vi "DSF.Engine.Framework.Rx.Async.vi"(8 "error in (no error)":errorcluster, 11 "Framework in":refnum<class "DSF.Engine.Framework.lvclass">) -> (0 "error out":errorcluster, 3 "Framework out":refnum<class "DSF.Engine.Framework.lvclass">)   [LabVIEW 2017, in "DSF.Engine.lvlib" / "DSF.Engine.Framework.lvclass"]
uses:
  DSF.Engine.Framework.lvclass
  DSF.Engine.Framework.lvclass/DSF.Engine.Framework.ctl
  Plugin/DSF.Engine.Plugin.lvclass/DSF.Engine.Plugin.ctl
  Timing/DSF.Engine.Timing.lvclass/DSF.Engine.Timing.ctl
  Transfer/DSF.Engine.Transfer Group.lvclass/DSF.Engine.Transfer Group.ctl
  Transfer/DSF.Engine.Transfer.lvclass/DSF.Engine.Transfer.ctl
  <vilib>/National Instruments/Memory Manager/Classes/Pointer/Memory.Pointer.lvclass/Memory.Pointer.ctl
  Thread Pool/DSF.Engine.Pool.lvclass/DSF.Engine.Pool.ctl
  Transceiver/DSF.Engine.Transceiver Thread.lvclass/DSF.Engine.Transceiver Thread.ctl
  Interface/DSF.Engine.Interface.lvclass/DSF.Engine.Interface.ctl
  Plugin/DSF.Engine.Plugin.Get Async Rx Transfer Groups.vi
  Timing/DSF.Engine.Timing.Get Iteration.vi
  Plugin/DSF.Engine.Plugin.Get Timing.vi
  Transfer/DSF.Engine.Transfer Group.Is Active.vi
  Plugin/DSF.Engine.Plugin.Rx.Transfer Group.Send.vi
  Plugin/DSF.Engine.Plugin.Rx.Transfer Group.Retrieve Async.vi
  Plugin/DSF.Engine.Plugin.Transfer Group.Iteration.Increment.vi
  Plugin/DSF.Engine.Plugin.Rx.Transfer Group.Move Data.vi
  Plugin/DSF.Engine.Plugin.Set Async Rx Transfer Groups.vi
  Timing/DSF.Engine.Timing.Is Active Cycle.vi
  Transfer/DSF.Engine.Transfer Group.Get Timing.vi
  Plugin/DSF.Engine.Plugin.Transceiver Thread.Obtain.vi
  Transceiver/DSF.Engine.Transceiver Thread.Command.Transfer Group.vi
  Transfer/DSF.Engine.Transfer Group.Retrieve from FIFO.vi
  Transfer/DSF.Engine.Transfer Group.Increment Iteration.vi
  Transfer/DSF.Engine.Transfer Group.Move Channels to Engine.vi
  Timing/DSF.Engine.Timing.Get Decimation.vi
  Timing/DSF.Engine.Timing.Get Offset.vi
  Thread Pool/DSF.Engine.Pool.ID.Obtain ID from Pool.vi
  Plugin/DSF.Engine.Plugin.Get Thread ID Pool.vi
  Plugin/DSF.Engine.Plugin.Get Transceiver Thread.vi
  Transceiver/DSF.Engine.Transceiver Thread.Get Interface.vi
  Interface/DSF.Engine.Interface.Transceiver.Write.vi
  Interface/DSF.Engine.Interface.Transceiver.Write.Command.vi
  Transfer/DSF.Engine.Transfer Group.Get ID.vi
  Transfer/DSF.Engine.Transfer Group.Return FIFO.Read.vi
  Transfer/DSF.Engine.Transfer Group.Set Timing.vi
  Timing/DSF.Engine.Timing.Iteration.Increment.vi
  Transfer/DSF.Engine.Transfer Group.Get Transfers.vi
  <vilib>/National Instruments/Memory Manager/Classes/Pointer/Memory.Pointer.Copy All.vi
  Transfer/DSF.Engine.Transfer.Get Inline Buffer.vi
  Transfer/DSF.Engine.Transfer.Get Intermediate Buffer.vi
  Thread Pool/DSF.Engine.Pool.Read FIFO.vi
  Interface/DSF.Engine.Interface.RT FIFO.Write.16B.vi
  Interface/DSF.Engine.Interface.Get Command FIFO.vi
  Transfer/DSF.Engine.Transfer Group.Get Return FIFO.vi
  Timing/DSF.Engine.Timing.Set Iteration.vi
  <vilib>/National Instruments/Memory Manager/Classes/Pointer/Memory.Pointer.Get Size.vi
  <vilib>/National Instruments/Memory Manager/Classes/Pointer/Memory.Pointer.Copy.vi
  Thread Pool/DSF.Engine.Pool.Get FIFO.vi
  <vilib>/National Instruments/Memory Manager/Classes/Pointer/Memory.Pointer.Copy.No Check.vi
  <vilib>/National Instruments/Memory Manager/Classes/Pointer/Memory.Pointer.Parameter Check.Subset.vi
  <vilib>/National Instruments/Memory Manager/Classes/Pointer/Memory.Pointer.Parameter Check.Null Pointer.vi
  <vilib>/National Instruments/Memory Manager/Classes/Pointer/Memory.Pointer.Get Address.vi
  <vilib>/National Instruments/Memory Manager/Classes/Pointer/Memory.Pointer.Errors.vi
  <vilib>/National Instruments/Memory Manager/Classes/Pointer/Memory.Pointer.Errors.Out of Bounds.vi
  <vilib>/National Instruments/Memory Manager/Classes/Pointer/Memory.Pointer.Errors.Null Pointer.vi
  <vilib>/NI/Static Error Handling/VIs/Static Error Handling.Source Buffer.Write.String.vi
  <vilib>/National Instruments/Memory Manager/Classes/Pointer/Memory.Pointer.Errors.Write Pointer Size.vi
  <vilib>/National Instruments/Memory Manager/Classes/Pointer/Memory.Pointer.Errors.Create Error.vi
  <vilib>/NI/Static Error Handling/VIs/Static Error Handling.Source Buffer.Write.Numeric.Scalar.Base10.vi
  <vilib>/NI/Static Error Handling/VIs/Static Error Handling.Source Buffer.Write.Numeric.Scalar.Base10 (U64).vi
  <vilib>/NI/Static Error Handling/VIs/Static Error Handling.Error Cluster Constant.vi
  <vilib>/NI/Static Error Handling/VIs/Static Error Handling.Error Cluster Constant (512B).vi
  <vilib>/NI/Static Error Handling/VIs/Static Error Handling.Parameters.Status.Set.vi
  <vilib>/NI/Static Error Handling/VIs/Static Error Handling.Parameters.Code.Set.vi
  <vilib>/NI/Static Error Handling/VIs/Static Error Handling.Parameters.VI Source.Set.vi
  <vilib>/National Instruments/Memory Manager/Constants/Memory.Constants.vi
  <vilib>/National Instruments/Memory Manager/Constants/Memory.Constants.Library Name.vi
  <vilib>/National Instruments/Memory Manager/Classes/Pointer/Memory.Pointer.Errors.Get Info.vi
  Pointer/DSF.Engine.Pointer.DBL.lvclass
  C:/Program Files (x86)/National Instruments/LabVIEW 2017/vi.lib/National Instruments/Memory Manager/Classes/Pointer/Memory.Pointer.lvclass
  Thread Pool/DSF.Engine.Pool.ID.lvclass
  C:/Git/DSF/Source/Engine/Classes/Thread Pool/DSF.Engine.Pool.lvclass
  Interface/DSF.Engine.Interface.Transceiver.lvclass
  C:/Git/DSF/Source/Engine/Classes/Interface/DSF.Engine.Interface.lvclass
  Transceiver/DSF.Engine.Transceiver Thread.lvclass
  Plugin/DSF.Engine.Plugin.lvclass
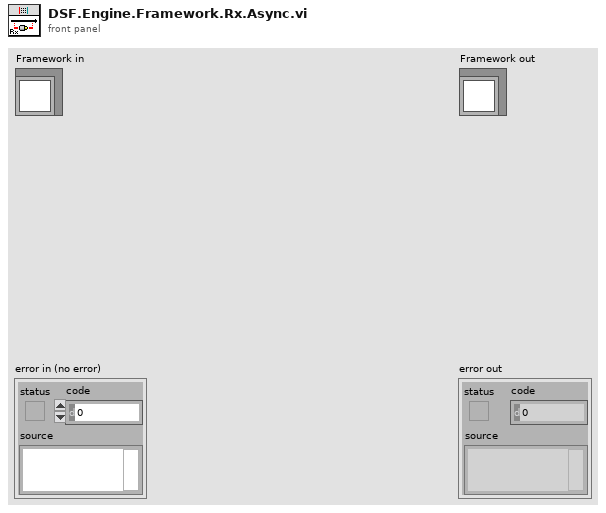
[diagram p1: front panel]
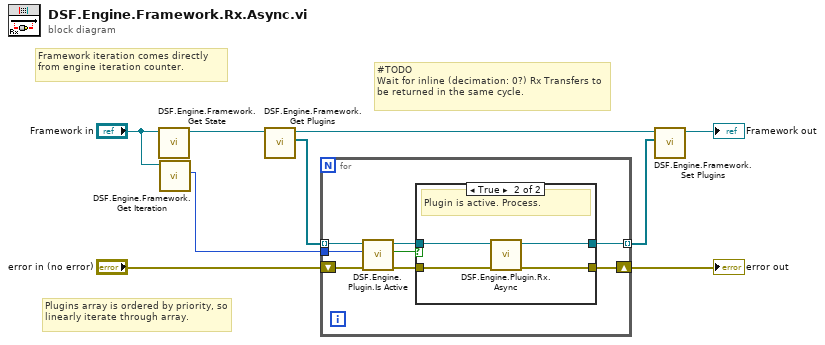
[diagram p0: block diagram]
diagram:
  # "#TODO\nWait for inline (decimation: 0?) Rx Transfers to be returned in the same cycle."
  # "Framework iteration comes directly from engine iteration counter."
  # "Plugins array is ordered by priority, so linearly iterate through array."
  n1 = call "DSF.Engine.Framework.Get State.vi"("Framework in"="Framework in") -> ("Framework out"=w4:refnum<class "DSF.Engine.Framework.lvclass">)  [unwired: 9 in, 1 out]
  n2 = call "DSF.Engine.Framework.Get Iteration.vi"("Framework in"="Framework in") -> ("iteration"=w2:u64)  [unwired: 9 in, 1 out]
  n3 = call "DSF.Engine.Framework.Get Plugins.vi"("Framework in"=w4) -> ("Plugins"=w9:refnum<class "DSF.Engine.Plugin.lvclass">[], "Framework out"=w5:refnum<class "DSF.Engine.Framework.lvclass">)  [unwired: 9 in]
  n4 = for {
    tunnel: w9 -> [w11] mode=indexing
    tunnel: [w16] -> w1 mode=indexing
    shift-right: [w15] -> w6
    shift-left: "error in (no error)" -> [w14]
    tunnel: w2 -> [w12]
    n5 = call "DSF.Engine.Plugin.Is Active.vi"("cycle count"=w12, "Plugin in"=w11) -> ("active this cycle?"=w10:bool, "Plugin out"=w13:refnum<class "DSF.Engine.Plugin.lvclass">)  [unwired: 8 in]
    n6 = case shown="True" w10 {
      tunnel: w13 -> [w18 w22]
      tunnel: [w18 w20] -> w16
      tunnel: [w17 w19] -> w15
      tunnel: w14 -> [w17 w21]
      frame False {
        # "Plugin is not active. Skip."
      }
      frame True {
        # "Plugin is active. Process."
        n7 = call "DSF.Engine.Plugin.Rx.Async.vi"("error in (no error)"=w21, "Plugin in"=w22) -> ("error out"=w19:errorcluster, "Plugin out"=w20:refnum<class "DSF.Engine.Plugin.lvclass">)  [unwired: 8 in]
      }
    }
  }
  "error out" <- w6
  n8 = call "DSF.Engine.Framework.Set Plugins.vi"("Plugins"=w1, "Framework in"=w5) -> ("Framework out"=→"Framework out":refnum<class "DSF.Engine.Framework.lvclass">)  [unwired: 9 in]
